vi "输入数据解析.vi"(0 "单个参数补充":dbl, 1 "从板号":dbl=1.0, 2 "主板二维码":string="BNET01", 3 "从板二维码":string="BNET01", 5 "主板引用":refnum<vi>, 7 "从板引用":refnum<vi>, 9 "主板选项":string="三级故障阀值", 11 "枚举":enum16{"主板", "从板"}(ring), 12 "快换":bool caption="快换写入") -> (4 "输出数组":dbl[][](array[numeric]), 6 "数组长度":dbl[](array[numeric]), 8 "循环次数":i32, 10 "命令":u32, 14 "名称":string[](array[string]), 15 "命令序号":u32[](array[numeric]))   [LabVIEW 2013] (continued)
                n2887 = Build Array(w7428, w7426) -> (w7429:i32[])
              }
            }
            n2888 = Insert Into Array(array=w7234, new element=w7235) -> (w7233:dbl[])  [unwired: 1 in]
          }
          n2889 = Build Array(w7230) -> (w7229:dbl[][])
          n2890 = Build Array("一级故障阀值") -> (w7220:string[])
        }
        frame "充电电流过高(2)" {
          n2891 = Unbundle By Name(w7455) -> ("一级故障 2"=w7456:refnum<vi>)
          n2892 = property class="Clust (严格)"(reference=w7456) -> ("Value"=w7454:T4)  [unwired: 1 in, 2 out]
          n2893 = for {
            N: 17 -> [_]
            tunnel: w7454 -> [w7466]
            shift-right: [w7463] -> w7460
            shift-left: dbl[] [] -> [w7464]
            i -> [w7467]
            n2894 = case shown="13" w7467 {
              tunnel: w7466 -> [w7468 w7479 w7490 w7500 w7510 w7520 w7532 w7544 w7556 w7568 w7580 w7592 w7606 w7627 w7639 w7648 w7657]
              tunnel: [w7469 w7480 w7491 w7501 w7511 w7522 w7534 w7546 w7558 w7570 w7582 w7593 w7615 w7630 w7638 w7647 w7659] -> w7465
              frame 0, Default {
                # "总电压过高"
                n2895 = disable-structure shown="启用" {
                  disable-tunnel: [w7475 w7478] -> w7471
                  disable-tunnel: [w7474 w7478] -> w7470
                  disable-tunnel: w7468 -> [w7473 _]
                  frame Disabled {
                    n2896 = Unbundle By Name(w7473) -> ("总电压过高"=w7472:dbl)
                    n2897 = call "输入分辨率计算-EV05.vi"("1字节?"=FALSE, "数值"=w7472, "分辨率"=0.1) -> ("低字节"=w7475:dbl, "高字节1"=w7474:dbl)  [unwired: 2 in, 5 out]
                  }
                  frame Enabled {
                    w7478 = 255 ("高字节1")
                  }
                }
                n2898 = Build Array(w7470, w7471) -> (w7469:i32[])
              }
              frame 1 {
                # "总电压过低"
                n2899 = disable-structure shown="启用" {
                  disable-tunnel: [w7486 w7489] -> w7482
                  disable-tunnel: [w7485 w7489] -> w7481
                  disable-tunnel: w7479 -> [w7484 _]
                  frame Disabled {
                    n2900 = Unbundle By Name(w7484) -> ("总电压过低"=w7483:dbl)
                    n2901 = call "输入分辨率计算-EV05.vi"("1字节?"=FALSE, "数值"=w7483, "分辨率"=0.1) -> ("低字节"=w7486:dbl, "高字节1"=w7485:dbl)  [unwired: 2 in, 5 out]
                  }
                  frame Enabled {
                    w7489 = 255 ("高字节1")
                  }
                }
                n2902 = Build Array(w7481, w7482) -> (w7480:i32[])
              }
              frame 2 {
                # "温度过高"
                n2903 = disable-structure shown="启用" {
                  disable-tunnel: [w7496 255 ("高字节1")] -> w7492
                  disable-tunnel: w7490 -> [w7494 _]
                  frame Disabled {
                    n2904 = Unbundle By Name(w7494) -> ("温度过高"=w7493:dbl)
                    n2905 = call "输入分辨率计算-EV05.vi"("1字节?"=TRUE, "数值"=w7493, "偏移量"=-40.0, "分辨率"=1.0) -> ("高字节1"=w7496:dbl)  [unwired: 1 in, 6 out]
                  }
                  frame Enabled {
                  }
                }
                n2906 = Build Array(w7492) -> (w7491:i32[])
              }
              frame 3 {
                # "温度过低"
                n2907 = disable-structure shown="启用" {
                  disable-tunnel: [w7506 255 ("高字节1")] -> w7502
                  disable-tunnel: w7500 -> [w7504 _]
                  frame Disabled {
                    n2908 = Unbundle By Name(w7504) -> ("温度过低"=w7503:dbl)
                    n2909 = call "输入分辨率计算-EV05.vi"("1字节?"=TRUE, "数值"=w7503, "偏移量"=-40.0, "分辨率"=1.0) -> ("高字节1"=w7506:dbl)  [unwired: 1 in, 6 out]
                  }
                  frame Enabled {
                  }
                }
                n2910 = Build Array(w7502) -> (w7501:i32[])
              }
              frame 4 {
                # "整组温度不均衡"
                n2911 = disable-structure shown="启用" {
                  disable-tunnel: [w7516 255 ("高字节1")] -> w7512
                  disable-tunnel: w7510 -> [w7514 _]
                  frame Disabled {
                    n2912 = Unbundle By Name(w7514) -> ("整组温度不均衡"=w7513:dbl)
                    n2913 = call "输入分辨率计算-EV05.vi"("1字节?"=TRUE, "数值"=w7513, "偏移量"=0.0, "分辨率"=1.0) -> ("高字节1"=w7516:dbl)  [unwired: 1 in, 6 out]
                  }
                  frame Enabled {
                  }
                }
                n2914 = Build Array(w7512) -> (w7511:i32[])
              }
              frame 5 {
                # "单组电压不均衡"
                n2915 = disable-structure shown="启用" {
                  disable-tunnel: [w7528 w7531] -> w7523
                  disable-tunnel: [w7526 w7531] -> w7521
                  disable-tunnel: w7520 -> [w7525 _]
                  frame Disabled {
                    n2916 = Unbundle By Name(w7525) -> ("单组电压不均衡"=w7524:dbl)
                    n2917 = call "输入分辨率计算-EV05.vi"("1字节?"=FALSE, "数值"=w7524, "偏移量"=0.0, "分辨率"=0.001) -> ("低字节"=w7526:dbl, "高字节1"=w7528:dbl)  [unwired: 1 in, 5 out]
                  }
                  frame Enabled {
                    w7531 = 255 ("高字节1")
                  }
                }
                n2918 = Build Array(w7523, w7521) -> (w7522:i32[])
              }
              frame 6 {
                # "整组电压不均衡"
                n2919 = disable-structure shown="启用" {
                  disable-tunnel: [w7540 w7543] -> w7535
                  disable-tunnel: [w7538 w7543] -> w7533
                  disable-tunnel: w7532 -> [w7537 _]
                  frame Disabled {
                    n2920 = Unbundle By Name(w7537) -> ("整组电压不均衡"=w7536:dbl)
                    n2921 = call "输入分辨率计算-EV05.vi"("1字节?"=FALSE, "数值"=w7536, "偏移量"=0.0, "分辨率"=0.001) -> ("低字节"=w7538:dbl, "高字节1"=w7540:dbl)  [unwired: 1 in, 5 out]
                  }
                  frame Enabled {
                    w7543 = 255 ("高字节1")
                  }
                }
                n2922 = Build Array(w7535, w7533) -> (w7534:i32[])
              }
              frame 7 {
                # "单体电压过高"
                n2923 = disable-structure shown="启用" {
                  disable-tunnel: [w7552 w7555] -> w7547
                  disable-tunnel: [w7550 w7555] -> w7545
                  disable-tunnel: w7544 -> [w7549 _]
                  frame Disabled {
                    n2924 = Unbundle By Name(w7549) -> ("单体电压过高"=w7548:dbl)
                    n2925 = call "输入分辨率计算-EV05.vi"("1字节?"=FALSE, "数值"=w7548, "偏移量"=0.0, "分辨率"=0.001) -> ("低字节"=w7550:dbl, "高字节1"=w7552:dbl)  [unwired: 1 in, 5 out]
                  }
                  frame Enabled {
                    w7555 = 255 ("高字节1")
                  }
                }
                n2926 = Build Array(w7547, w7545) -> (w7546:i32[])
              }
              frame 8 {
                # "单体电压过低"
                n2927 = disable-structure shown="启用" {
                  disable-tunnel: [w7564 w7567] -> w7559
                  disable-tunnel: [w7562 w7567] -> w7557
                  disable-tunnel: w7556 -> [w7561 _]
                  frame Disabled {
                    n2928 = Unbundle By Name(w7561) -> ("单体电压过低"=w7560:dbl)
                    n2929 = call "输入分辨率计算-EV05.vi"("1字节?"=FALSE, "数值"=w7560, "偏移量"=0.0, "分辨率"=0.001) -> ("低字节"=w7562:dbl, "高字节1"=w7564:dbl)  [unwired: 1 in, 5 out]
                  }
                  frame Enabled {
                    w7567 = 255 ("高字节1")
                  }
                }
                n2930 = Build Array(w7559, w7557) -> (w7558:i32[])
              }
              frame 9 {
                # "充电电流过高"
                n2931 = disable-structure shown="启用" {
                  disable-tunnel: [w7576 w7579] -> w7571
                  disable-tunnel: [w7574 w7579] -> w7569
                  disable-tunnel: w7568 -> [w7573 _]
                  frame Enabled {
                    n2932 = Unbundle By Name(w7573) -> ("充电电流过高"=w7572:dbl)
                    n2933 = call "输入分辨率计算-EV05.vi"("1字节?"=FALSE, "数值"=w7572, "偏移量"=0.0, "分辨率"=0.1) -> ("低字节"=w7574:dbl, "高字节1"=w7576:dbl)  [unwired: 1 in, 5 out]
                  }
                  frame Disabled {
                    w7579 = 255 ("高字节1")
                  }
                }
                n2934 = Build Array(w7571, w7569) -> (w7570:dbl[])
              }
              frame 10 {
                # "放电电流过高"
                n2935 = disable-structure shown="启用" {
                  disable-tunnel: [w7588 w7591] -> w7583
                  disable-tunnel: [w7586 w7591] -> w7581
                  disable-tunnel: w7580 -> [w7585 _]
                  frame Disabled {
                    n2936 = Unbundle By Name(w7585) -> ("放电电流过高"=w7584:dbl)
                    n2937 = call "输入分辨率计算-EV05.vi"("1字节?"=FALSE, "数值"=w7584, "偏移量"=-3000.0, "分辨率"=0.1) -> ("低字节"=w7586:dbl, "高字节1"=w7588:dbl)  [unwired: 1 in, 5 out]
                  }
                  frame Enabled {
                    w7591 = 255 ("高字节1")
                  }
                }
                n2938 = Build Array(w7583, w7581) -> (w7582:i32[])
              }
              frame 11 {
                # "单组温度不均衡"
                n2939 = disable-structure shown="启用" {
                  disable-tunnel: [w7598 255 ("高字节1")] -> w7594
                  disable-tunnel: w7592 -> [w7596 _]
                  frame Disabled {
                    n2940 = Unbundle By Name(w7596) -> ("单组温度不均衡"=w7595:dbl)
                    n2941 = call "输入分辨率计算-EV05.vi"("1字节?"=TRUE, "数值"=w7595, "偏移量"=0.0, "分辨率"=1.0) -> ("高字节1"=w7598:dbl)  [unwired: 1 in, 6 out]
                  }
                  frame Enabled {
                  }
                }
                n2942 = Build Array(w7594) -> (w7593:i32[])
              }
              frame 12 {
                # "SOC过高"
                n2943 = Unbundle By Name(w7606) -> ("SOC过高"=w7605:dbl)
                n2944 = call "输入分辨率计算-EV05.vi"("1字节?"=FALSE, "数值"=w7605, "偏移量"=0.0, "分辨率"=0.1) -> ("低字节"=w7607:dbl, "高字节1"=w7608:dbl)  [unwired: 1 in, 5 out]
                n2945 = call "二进制解析-8.6.vi"("索引"=4, "数值"=w7608) -> ("低位子数组"=w7611:i32[])  [unwired: 3 out]
                n2946 = call "二进制解析-8.6.vi"("索引"=4, "数值"=w7607) -> ("低位子数组"=w7603:i32[], "高位子数组"=w7610:i32[])  [unwired: 2 out]
                n2947 = Insert Into Array(array=w7611, new element=w7610) -> (w7609:i32[])  [unwired: 1 in]
                n2948 = call "数值二进制转十进制-8.6.vi"("子数组"=w7609) -> ("十进制数值"=w7604:i32)  [unwired: 4 out]
                n2949 = disable-structure shown="启用" {
                  disable-tunnel: w7604 -> [w7619 _]
                  disable-tunnel: [w7619 255 ("高字节1")] -> w7602
                  disable-tunnel: [w7618 i32[] [] ("低位子数组 27")] -> _
                  disable-tunnel: w7603 -> [w7618 _]
                  frame Disabled {
                  }
                  frame Enabled {
                  }
                }
                n2950 = Build Array(w7602, w7602) -> (w7615:i32[])
              }
              frame 13 {
                # "SOC过低"
                n2951 = Unbundle By Name(w7627) -> ("SOC过低"=w7626:dbl)
                n2952 = call "输入分辨率计算-EV05.vi"("1字节?"=FALSE, "数值"=w7626, "偏移量"=0.0, "分辨率"=0.1) -> ("低字节"=w7624:dbl, "高字节1"=w7625:dbl)  [unwired: 1 in, 5 out]
                n2953 = call "二进制解析-8.6.vi"("索引"=4, "数值"=w7625) -> ("低位子数组"=w7623:i32[])  [unwired: 3 out]
                n2954 = disable-structure shown="启用" {
                  disable-tunnel: w7624 -> [w7634 _]
                  disable-tunnel: [w7634 255 ("高字节1")] -> w7622
                  disable-tunnel: w7623 -> [w7633 _]
                  disable-tunnel: [w7633 i32[] [] ("低位子数组")] -> _
                  frame Disabled {
                    (unwired) i32[] [] ("低位子数组 4")
                  }
                  frame Enabled {
                  }
                }
                n2955 = Build Array(w7622, w7622) -> (w7630:i32[])
              }
              frame 14 {
                # "内阻过大"
                n2956 = disable-structure shown="启用" {
                  disable-tunnel: w7639 -> [w7644 _]
                  disable-tunnel: [w7640 255 ("高字节1")] -> w7637
                  frame Disabled {
                    n2957 = Unbundle By Name(w7644) -> ("内阻过大"=w7643:dbl)
                    n2958 = call "输入分辨率计算-EV05.vi"("1字节?"=TRUE, "数值"=w7643, "分辨率"=0.1) -> ("高字节1"=w7640:dbl)  [unwired: 2 in, 6 out]
                  }
                  frame Enabled {
                  }
                }
                n2959 = Build Array(w7637) -> (w7638:i32[])
              }
              frame 15 {
                # "极柱温度过高"
                n2960 = disable-structure shown="启用" {
                  disable-tunnel: w7648 -> [w7654 _]
                  disable-tunnel: [w7650 255 ("高字节1")] -> w7646
                  frame Disabled {
                    n2961 = Unbundle By Name(w7654) -> ("极柱温度过高"=w7653:dbl)
                    n2962 = call "输入分辨率计算-EV05.vi"("1字节?"=TRUE, "数值"=w7653, "偏移量"=-40.0, "分辨率"=1.0) -> ("高字节1"=w7650:dbl)  [unwired: 1 in, 6 out]
                  }
                  frame Enabled {
                  }
                }
                n2963 = Build Array(w7646) -> (w7647:i32[])
              }
              frame 16 {
                # "SOH过低"
                n2964 = disable-structure shown="启用" {
                  disable-tunnel: [w7671 w7679] -> w7658
                  disable-tunnel: w7657 -> [w7668 _]
                  disable-tunnel: [w7660 w7679] -> w7656
                  frame Disabled {
                    n2965 = Unbundle By Name(w7668) -> ("SOH过低"=w7667:dbl)
                    n2966 = call "输入分辨率计算-EV05.vi"("1字节?"=FALSE, "数值"=w7667, "偏移量"=0.0, "分辨率"=0.1) -> ("低字节"=w7669:dbl, "高字节1"=w7670:dbl)  [unwired: 1 in, 5 out]
                    n2967 = call "二进制解析-8.6.vi"("索引"=4, "数值"=w7670) -> ("低位子数组"=w7673:i32[])  [unwired: 3 out]
                    n2968 = call "二进制解析-8.6.vi"("索引"=4, "数值"=w7669) -> ("低位子数组"=w7662:i32[], "高位子数组"=w7672:i32[])  [unwired: 2 out]
                    n2969 = call "二进制解析-8.6.vi"("索引"=4, "数值"=0) -> ("低位子数组"=w7663:i32[])  [unwired: 3 out]
                    n2970 = Insert Into Array(array=w7673, new element=w7672) -> (w7666:i32[])  [unwired: 1 in]
                    n2971 = Insert Into Array(array=w7662, new element=w7663) -> (w7661:i32[])  [unwired: 1 in]
                    n2972 = call "数值二进制转十进制-8.6.vi"("子数组"=w7666) -> ("十进制数值"=w7671:i32)  [unwired: 4 out]
                    n2973 = call "数值二进制转十进制-8.6.vi"("子数组"=w7661) -> ("十进制数值"=w7660:i32)  [unwired: 4 out]
                  }
                  frame Enabled {
                    w7679 = 255 ("高字节1")
                  }
                }
                n2974 = Build Array(w7658, w7656) -> (w7659:i32[])
              }
            }
            n2975 = Insert Into Array(array=w7464, new element=w7465) -> (w7463:dbl[])  [unwired: 1 in]
          }
          n2976 = Build Array(w7460) -> (w7459:dbl[][])
          n2977 = Build Array("二级故障阀值") -> (w7450:string[])
        }
        frame "充电电流过高(3)" {
          n2978 = Unbundle By Name(w7685) -> ("一级故障 3"=w7686:refnum<vi>)
          n2979 = property class="Clust (严格)"(reference=w7686) -> ("Value"=w7684:T4)  [unwired: 1 in, 2 out]
          n2980 = for {
            N: 17 -> [_]
            tunnel: w7684 -> [w7696]
            shift-right: [w7693] -> w7690
            shift-left: dbl[] [] -> [w7694]
            i -> [w7697]
            n2981 = case shown="13" w7697 {
              tunnel: w7696 -> [w7698 w7709 w7720 w7730 w7740 w7750 w7762 w7774 w7786 w7798 w7810 w7822 w7836 w7857 w7869 w7878 w7887]
              tunnel: [w7699 w7710 w7721 w7731 w7741 w7752 w7764 w7776 w7788 w7800 w7812 w7823 w7845 w7860 w7868 w7877 w7889] -> w7695
              frame 0, Default {
                # "总电压过高"
                n2982 = disable-structure shown="启用" {
                  disable-tunnel: [w7705 w7708] -> w7701
                  disable-tunnel: [w7704 w7708] -> w7700
                  disable-tunnel: w7698 -> [w7703 _]
                  frame Disabled {
                    n2983 = Unbundle By Name(w7703) -> ("总电压过高"=w7702:dbl)
                    n2984 = call "输入分辨率计算-EV05.vi"("1字节?"=FALSE, "数值"=w7702, "分辨率"=0.1) -> ("低字节"=w7705:dbl, "高字节1"=w7704:dbl)  [unwired: 2 in, 5 out]
                  }
                  frame Enabled {
                    w7708 = 255 ("高字节1")
                  }
                }
                n2985 = Build Array(w7700, w7701) -> (w7699:i32[])
              }
              frame 1 {
                # "总电压过低"
                n2986 = disable-structure shown="启用" {
                  disable-tunnel: [w7716 w7719] -> w7712
                  disable-tunnel: [w7715 w7719] -> w7711
                  disable-tunnel: w7709 -> [w7714 _]
                  frame Disabled {
                    n2987 = Unbundle By Name(w7714) -> ("总电压过低"=w7713:dbl)
                    n2988 = call "输入分辨率计算-EV05.vi"("1字节?"=FALSE, "数值"=w7713, "分辨率"=0.1) -> ("低字节"=w7716:dbl, "高字节1"=w7715:dbl)  [unwired: 2 in, 5 out]
                  }
                  frame Enabled {
                    w7719 = 255 ("高字节1")
                  }
                }
                n2989 = Build Array(w7711, w7712) -> (w7710:i32[])
              }
              frame 2 {
                # "温度过高"
                n2990 = disable-structure shown="启用" {
                  disable-tunnel: [w7726 255 ("高字节1")] -> w7722
                  disable-tunnel: w7720 -> [w7724 _]
                  frame Disabled {
                    n2991 = Unbundle By Name(w7724) -> ("温度过高"=w7723:dbl)
                    n2992 = call "输入分辨率计算-EV05.vi"("1字节?"=TRUE, "数值"=w7723, "偏移量"=-40.0, "分辨率"=1.0) -> ("高字节1"=w7726:dbl)  [unwired: 1 in, 6 out]
                  }
                  frame Enabled {
                  }
                }
                n2993 = Build Array(w7722) -> (w7721:i32[])
              }
              frame 3 {
                # "温度过低"
                n2994 = disable-structure shown="启用" {
                  disable-tunnel: [w7736 255 ("高字节1")] -> w7732
                  disable-tunnel: w7730 -> [w7734 _]
                  frame Disabled {
                    n2995 = Unbundle By Name(w7734) -> ("温度过低"=w7733:dbl)
                    n2996 = call "输入分辨率计算-EV05.vi"("1字节?"=TRUE, "数值"=w7733, "偏移量"=-40.0, "分辨率"=1.0) -> ("高字节1"=w7736:dbl)  [unwired: 1 in, 6 out]
                  }
                  frame Enabled {
                  }
                }
                n2997 = Build Array(w7732) -> (w7731:i32[])
              }
              frame 4 {
                # "整组温度不均衡"
                n2998 = disable-structure shown="启用" {
                  disable-tunnel: [w7746 255 ("高字节1")] -> w7742
                  disable-tunnel: w7740 -> [w7744 _]
                  frame Disabled {
                    n2999 = Unbundle By Name(w7744) -> ("整组温度不均衡"=w7743:dbl)
                    n3000 = call "输入分辨率计算-EV05.vi"("1字节?"=TRUE, "数值"=w7743, "偏移量"=0.0, "分辨率"=1.0) -> ("高字节1"=w7746:dbl)  [unwired: 1 in, 6 out]
                  }
                  frame Enabled {
                  }
                }
                n3001 = Build Array(w7742) -> (w7741:i32[])
              }
              frame 5 {
                # "单组电压不均衡"
                n3002 = disable-structure shown="启用" {
                  disable-tunnel: [w7758 w7761] -> w7753
                  disable-tunnel: [w7756 w7761] -> w7751
                  disable-tunnel: w7750 -> [w7755 _]
                  frame Disabled {
                    n3003 = Unbundle By Name(w7755) -> ("单组电压不均衡"=w7754:dbl)
                    n3004 = call "输入分辨率计算-EV05.vi"("1字节?"=FALSE, "数值"=w7754, "偏移量"=0.0, "分辨率"=0.001) -> ("低字节"=w7756:dbl, "高字节1"=w7758:dbl)  [unwired: 1 in, 5 out]
                  }
                  frame Enabled {
                    w7761 = 255 ("高字节1")
                  }
                }
                n3005 = Build Array(w7753, w7751) -> (w7752:i32[])
              }
              frame 6 {
                # "整组电压不均衡"
                n3006 = disable-structure shown="启用" {
                  disable-tunnel: [w7770 w7773] -> w7765
                  disable-tunnel: [w7768 w7773] -> w7763
                  disable-tunnel: w7762 -> [w7767 _]
                  frame Disabled {
                    n3007 = Unbundle By Name(w7767) -> ("整组电压不均衡"=w7766:dbl)
                    n3008 = call "输入分辨率计算-EV05.vi"("1字节?"=FALSE, "数值"=w7766, "偏移量"=0.0, "分辨率"=0.001) -> ("低字节"=w7768:dbl, "高字节1"=w7770:dbl)  [unwired: 1 in, 5 out]
                  }
                  frame Enabled {
                    w7773 = 255 ("高字节1")
                  }
                }
                n3009 = Build Array(w7765, w7763) -> (w7764:i32[])
              }
              frame 7 {
                # "单体电压过高"
                n3010 = disable-structure shown="启用" {
                  disable-tunnel: [w7782 w7785] -> w7777
                  disable-tunnel: [w7780 w7785] -> w7775
                  disable-tunnel: w7774 -> [w7779 _]
                  frame Disabled {
                    n3011 = Unbundle By Name(w7779) -> ("单体电压过高"=w7778:dbl)
                    n3012 = call "输入分辨率计算-EV05.vi"("1字节?"=FALSE, "数值"=w7778, "偏移量"=0.0, "分辨率"=0.001) -> ("低字节"=w7780:dbl, "高字节1"=w7782:dbl)  [unwired: 1 in, 5 out]
                  }
                  frame Enabled {
                    w7785 = 255 ("高字节1")
                  }
                }
                n3013 = Build Array(w7777, w7775) -> (w7776:i32[])
              }
              frame 8 {
                # "单体电压过低"
                n3014 = disable-structure shown="启用" {
                  disable-tunnel: [w7794 w7797] -> w7789
                  disable-tunnel: [w7792 w7797] -> w7787
                  disable-tunnel: w7786 -> [w7791 _]
                  frame Disabled {
                    n3015 = Unbundle By Name(w7791) -> ("单体电压过低"=w7790:dbl)
                    n3016 = call "输入分辨率计算-EV05.vi"("1字节?"=FALSE, "数值"=w7790, "偏移量"=0.0, "分辨率"=0.001) -> ("低字节"=w7792:dbl, "高字节1"=w7794:dbl)  [unwired: 1 in, 5 out]
                  }
                  frame Enabled {
                    w7797 = 255 ("高字节1")
                  }
                }
                n3017 = Build Array(w7789, w7787) -> (w7788:i32[])
              }
              frame 9 {
                # "充电电流过高"
                n3018 = disable-structure shown="启用" {
                  disable-tunnel: [w7806 w7809] -> w7801
                  disable-tunnel: [w7804 w7809] -> w7799
                  disable-tunnel: w7798 -> [w7803 _]
                  frame Enabled {
                    n3019 = Unbundle By Name(w7803) -> ("充电电流过高"=w7802:dbl)
                    n3020 = call "输入分辨率计算-EV05.vi"("1字节?"=FALSE, "数值"=w7802, "偏移量"=0.0, "分辨率"=0.1) -> ("低字节"=w7804:dbl, "高字节1"=w7806:dbl)  [unwired: 1 in, 5 out]
                  }
                  frame Disabled {
                    w7809 = 255 ("高字节1")
                  }
                }
                n3021 = Build Array(w7801, w7799) -> (w7800:dbl[])
              }
              frame 10 {
                # "放电电流过高"
                n3022 = disable-structure shown="启用" {
                  disable-tunnel: [w7818 w7821] -> w7813
                  disable-tunnel: [w7816 w7821] -> w7811
                  disable-tunnel: w7810 -> [w7815 _]
                  frame Disabled {
                    n3023 = Unbundle By Name(w7815) -> ("放电电流过高"=w7814:dbl)
                    n3024 = call "输入分辨率计算-EV05.vi"("1字节?"=FALSE, "数值"=w7814, "偏移量"=-3000.0, "分辨率"=0.1) -> ("低字节"=w7816:dbl, "高字节1"=w7818:dbl)  [unwired: 1 in, 5 out]
                  }
                  frame Enabled {
                    w7821 = 255 ("高字节1")
                  }
                }
                n3025 = Build Array(w7813, w7811) -> (w7812:i32[])
              }
              frame 11 {
                # "单组温度不均衡"
                n3026 = disable-structure shown="启用" {
                  disable-tunnel: [w7828 255 ("高字节1")] -> w7824
                  disable-tunnel: w7822 -> [w7826 _]
                  frame Disabled {
                    n3027 = Unbundle By Name(w7826) -> ("单组温度不均衡"=w7825:dbl)
                    n3028 = call "输入分辨率计算-EV05.vi"("1字节?"=TRUE, "数值"=w7825, "偏移量"=0.0, "分辨率"=1.0) -> ("高字节1"=w7828:dbl)  [unwired: 1 in, 6 out]
                  }
                  frame Enabled {
                  }
                }
                n3029 = Build Array(w7824) -> (w7823:i32[])
              }
              frame 12 {
                # "SOC过高"
                n3030 = Unbundle By Name(w7836) -> ("SOC过高"=w7835:dbl)
                n3031 = call "输入分辨率计算-EV05.vi"("1字节?"=FALSE, "数值"=w7835, "偏移量"=0.0, "分辨率"=0.1) -> ("低字节"=w7837:dbl, "高字节1"=w7838:dbl)  [unwired: 1 in, 5 out]
                n3032 = call "二进制解析-8.6.vi"("索引"=4, "数值"=w7838) -> ("低位子数组"=w7841:i32[])  [unwired: 3 out]
                n3033 = call "二进制解析-8.6.vi"("索引"=4, "数值"=w7837) -> ("低位子数组"=w7833:i32[], "高位子数组"=w7840:i32[])  [unwired: 2 out]
                n3034 = Insert Into Array(array=w7841, new element=w7840) -> (w7839:i32[])  [unwired: 1 in]
                n3035 = call "数值二进制转十进制-8.6.vi"("子数组"=w7839) -> ("十进制数值"=w7834:i32)  [unwired: 4 out]
                n3036 = disable-structure shown="启用" {
                  disable-tunnel: w7834 -> [w7849 _]
                  disable-tunnel: [w7849 255 ("高字节1")] -> w7832
                  disable-tunnel: [w7848 i32[] [] ("低位子数组 27")] -> _
                  disable-tunnel: w7833 -> [w7848 _]
                  frame Disabled {
                  }
                  frame Enabled {
                  }
                }
                n3037 = Build Array(w7832, w7832) -> (w7845:i32[])
              }
              frame 13 {
                # "SOC过低"
                n3038 = Unbundle By Name(w7857) -> ("SOC过低"=w7856:dbl)
                n3039 = call "输入分辨率计算-EV05.vi"("1字节?"=FALSE, "数值"=w7856, "偏移量"=0.0, "分辨率"=0.1) -> ("低字节"=w7854:dbl, "高字节1"=w7855:dbl)  [unwired: 1 in, 5 out]
                n3040 = call "二进制解析-8.6.vi"("索引"=4, "数值"=w7855) -> ("低位子数组"=w7853:i32[])  [unwired: 3 out]
                n3041 = disable-structure shown="启用" {
                  disable-tunnel: w7854 -> [w7864 _]
                  disable-tunnel: [w7864 255 ("高字节1")] -> w7852
                  disable-tunnel: w7853 -> [w7863 _]
                  disable-tunnel: [w7863 i32[] [] ("低位子数组")] -> _
                  frame Disabled {
                    (unwired) i32[] [] ("低位子数组 4")
                  }
                  frame Enabled {
                  }
                }
                n3042 = Build Array(w7852, w7852) -> (w7860:i32[])
              }
              frame 14 {
                # "内阻过大"
                n3043 = disable-structure shown="启用" {
                  disable-tunnel: w7869 -> [w7874 _]
                  disable-tunnel: [w7870 255 ("高字节1")] -> w7867
                  frame Disabled {
                    n3044 = Unbundle By Name(w7874) -> ("内阻过大"=w7873:dbl)
                    n3045 = call "输入分辨率计算-EV05.vi"("1字节?"=TRUE, "数值"=w7873, "分辨率"=0.1) -> ("高字节1"=w7870:dbl)  [unwired: 2 in, 6 out]
                  }
                  frame Enabled {
                  }
                }
                n3046 = Build Array(w7867) -> (w7868:i32[])
              }
              frame 15 {
                # "极柱温度过高"
                n3047 = disable-structure shown="启用" {
                  disable-tunnel: w7878 -> [w7884 _]
                  disable-tunnel: [w7880 255 ("高字节1")] -> w7876
                  frame Disabled {
                    n3048 = Unbundle By Name(w7884) -> ("极柱温度过高"=w7883:dbl)
                    n3049 = call "输入分辨率计算-EV05.vi"("1字节?"=TRUE, "数值"=w7883, "偏移量"=-40.0, "分辨率"=1.0) -> ("高字节1"=w7880:dbl)  [unwired: 1 in, 6 out]
                  }
                  frame Enabled {
                  }
                }
                n3050 = Build Array(w7876) -> (w7877:i32[])
              }
              frame 16 {
                # "SOH过低"
                n3051 = disable-structure shown="启用" {
                  disable-tunnel: [w7901 w7909] -> w7888
                  disable-tunnel: w7887 -> [w7898 _]
                  disable-tunnel: [w7890 w7909] -> w7886
                  frame Disabled {
                    n3052 = Unbundle By Name(w7898) -> ("SOH过低"=w7897:dbl)
                    n3053 = call "输入分辨率计算-EV05.vi"("1字节?"=FALSE, "数值"=w7897, "偏移量"=0.0, "分辨率"=0.1) -> ("低字节"=w7899:dbl, "高字节1"=w7900:dbl)  [unwired: 1 in, 5 out]
                    n3054 = call "二进制解析-8.6.vi"("索引"=4, "数值"=w7900) -> ("低位子数组"=w7903:i32[])  [unwired: 3 out]
                    n3055 = call "二进制解析-8.6.vi"("索引"=4, "数值"=w7899) -> ("低位子数组"=w7892:i32[], "高位子数组"=w7902:i32[])  [unwired: 2 out]
                    n3056 = call "二进制解析-8.6.vi"("索引"=4, "数值"=0) -> ("低位子数组"=w7893:i32[])  [unwired: 3 out]
                    n3057 = Insert Into Array(array=w7903, new element=w7902) -> (w7896:i32[])  [unwired: 1 in]
                    n3058 = Insert Into Array(array=w7892, new element=w7893) -> (w7891:i32[])  [unwired: 1 in]
                    n3059 = call "数值二进制转十进制-8.6.vi"("子数组"=w7896) -> ("十进制数值"=w7901:i32)  [unwired: 4 out]
                    n3060 = call "数值二进制转十进制-8.6.vi"("子数组"=w7891) -> ("十进制数值"=w7890:i32)  [unwired: 4 out]
                  }
                  frame Enabled {
                    w7909 = 255 ("高字节1")
                  }
                }
                n3061 = Build Array(w7888, w7886) -> (w7889:i32[])
              }
            }
            n3062 = Insert Into Array(array=w7694, new element=w7695) -> (w7693:dbl[])  [unwired: 1 in]
          }
          n3063 = Build Array(w7690) -> (w7689:dbl[][])
          n3064 = Build Array("三级故障阀值") -> (w7680:string[])
        }
        frame "放电电流过高" {
          n3065 = Unbundle By Name(w7915) -> ("一级故障"=w7916:refnum<vi>)
          n3066 = property class="Clust (严格)"(reference=w7916) -> ("Value"=w7914:T4)  [unwired: 1 in, 2 out]
          n3067 = for {
            N: 17 -> [_]
            tunnel: w7914 -> [w7926]
            shift-right: [w7923] -> w7920
            shift-left: dbl[] [] -> [w7924]
            i -> [w7927]
            n3068 = case shown="14" w7927 {
              tunnel: w7926 -> [w7928 w7939 w7950 w7960 w7970 w7980 w7992 w8004 w8016 w8028 w8040 w8052 w8066 w8087 w8099 w8108 w8117]
              tunnel: [w7929 w7940 w7951 w7961 w7971 w7982 w7994 w8006 w8018 w8030 w8042 w8053 w8075 w8090 w8098 w8107 w8119] -> w7925
              frame 0, Default {
                # "总电压过高"
                n3069 = disable-structure shown="启用" {
                  disable-tunnel: [w7935 w7938] -> w7931
                  disable-tunnel: [w7934 w7938] -> w7930
                  disable-tunnel: w7928 -> [w7933 _]
                  frame Disabled {
                    n3070 = Unbundle By Name(w7933) -> ("总电压过高"=w7932:dbl)
                    n3071 = call "输入分辨率计算-EV05.vi"("1字节?"=FALSE, "数值"=w7932, "分辨率"=0.1) -> ("低字节"=w7935:dbl, "高字节1"=w7934:dbl)  [unwired: 2 in, 5 out]
                  }
                  frame Enabled {
                    w7938 = 255 ("高字节1")
                  }
                }
                n3072 = Build Array(w7930, w7931) -> (w7929:i32[])
              }
              frame 1 {
                # "总电压过低"
                n3073 = disable-structure shown="启用" {
                  disable-tunnel: [w7946 w7949] -> w7942
                  disable-tunnel: [w7945 w7949] -> w7941
                  disable-tunnel: w7939 -> [w7944 _]
                  frame Disabled {
                    n3074 = Unbundle By Name(w7944) -> ("总电压过低"=w7943:dbl)
                    n3075 = call "输入分辨率计算-EV05.vi"("1字节?"=FALSE, "数值"=w7943, "分辨率"=0.1) -> ("低字节"=w7946:dbl, "高字节1"=w7945:dbl)  [unwired: 2 in, 5 out]
                  }
                  frame Enabled {
                    w7949 = 255 ("高字节1")
                  }
                }
                n3076 = Build Array(w7941, w7942) -> (w7940:i32[])
              }
              frame 2 {
                # "温度过高"
                n3077 = disable-structure shown="启用" {
                  disable-tunnel: [w7956 255 ("高字节1")] -> w7952
                  disable-tunnel: w7950 -> [w7954 _]
                  frame Disabled {
                    n3078 = Unbundle By Name(w7954) -> ("温度过高"=w7953:dbl)
                    n3079 = call "输入分辨率计算-EV05.vi"("1字节?"=TRUE, "数值"=w7953, "偏移量"=-40.0, "分辨率"=1.0) -> ("高字节1"=w7956:dbl)  [unwired: 1 in, 6 out]
                  }
                  frame Enabled {
                  }
                }
                n3080 = Build Array(w7952) -> (w7951:i32[])
              }
              frame 3 {
                # "温度过低"
                n3081 = disable-structure shown="启用" {
                  disable-tunnel: [w7966 255 ("高字节1")] -> w7962
                  disable-tunnel: w7960 -> [w7964 _]
                  frame Disabled {
                    n3082 = Unbundle By Name(w7964) -> ("温度过低"=w7963:dbl)
                    n3083 = call "输入分辨率计算-EV05.vi"("1字节?"=TRUE, "数值"=w7963, "偏移量"=-40.0, "分辨率"=1.0) -> ("高字节1"=w7966:dbl)  [unwired: 1 in, 6 out]
                  }
                  frame Enabled {
                  }
                }
                n3084 = Build Array(w7962) -> (w7961:i32[])
              }
              frame 4 {
                # "整组温度不均衡"
                n3085 = disable-structure shown="启用" {
                  disable-tunnel: [w7976 255 ("高字节1")] -> w7972
                  disable-tunnel: w7970 -> [w7974 _]
                  frame Disabled {
                    n3086 = Unbundle By Name(w7974) -> ("整组温度不均衡"=w7973:dbl)
                    n3087 = call "输入分辨率计算-EV05.vi"("1字节?"=TRUE, "数值"=w7973, "偏移量"=0.0, "分辨率"=1.0) -> ("高字节1"=w7976:dbl)  [unwired: 1 in, 6 out]
                  }
                  frame Enabled {
                  }
                }
                n3088 = Build Array(w7972) -> (w7971:i32[])
              }
              frame 5 {
                # "单组电压不均衡"
                n3089 = disable-structure shown="启用" {
                  disable-tunnel: [w7988 w7991] -> w7983
                  disable-tunnel: [w7986 w7991] -> w7981
                  disable-tunnel: w7980 -> [w7985 _]
                  frame Disabled {
                    n3090 = Unbundle By Name(w7985) -> ("单组电压不均衡"=w7984:dbl)
                    n3091 = call "输入分辨率计算-EV05.vi"("1字节?"=FALSE, "数值"=w7984, "偏移量"=0.0, "分辨率"=0.001) -> ("低字节"=w7986:dbl, "高字节1"=w7988:dbl)  [unwired: 1 in, 5 out]
                  }
                  frame Enabled {
                    w7991 = 255 ("高字节1")
                  }
                }
                n3092 = Build Array(w7983, w7981) -> (w7982:i32[])
              }
              frame 6 {
                # "整组电压不均衡"
                n3093 = disable-structure shown="启用" {
                  disable-tunnel: [w8000 w8003] -> w7995
                  disable-tunnel: [w7998 w8003] -> w7993
                  disable-tunnel: w7992 -> [w7997 _]
                  frame Disabled {
                    n3094 = Unbundle By Name(w7997) -> ("整组电压不均衡"=w7996:dbl)
                    n3095 = call "输入分辨率计算-EV05.vi"("1字节?"=FALSE, "数值"=w7996, "偏移量"=0.0, "分辨率"=0.001) -> ("低字节"=w7998:dbl, "高字节1"=w8000:dbl)  [unwired: 1 in, 5 out]
                  }
                  frame Enabled {
                    w8003 = 255 ("高字节1")
                  }
                }
                n3096 = Build Array(w7995, w7993) -> (w7994:i32[])
              }
              frame 7 {
                # "单体电压过高"
                n3097 = disable-structure shown="启用" {
                  disable-tunnel: [w8012 w8015] -> w8007
                  disable-tunnel: [w8010 w8015] -> w8005
                  disable-tunnel: w8004 -> [w8009 _]
                  frame Disabled {
                    n3098 = Unbundle By Name(w8009) -> ("单体电压过高"=w8008:dbl)
                    n3099 = call "输入分辨率计算-EV05.vi"("1字节?"=FALSE, "数值"=w8008, "偏移量"=0.0, "分辨率"=0.001) -> ("低字节"=w8010:dbl, "高字节1"=w8012:dbl)  [unwired: 1 in, 5 out]
                  }
                  frame Enabled {
                    w8015 = 255 ("高字节1")
                  }
                }
                n3100 = Build Array(w8007, w8005) -> (w8006:i32[])
              }
              frame 8 {
                # "单体电压过低"
                n3101 = disable-structure shown="启用" {
                  disable-tunnel: [w8024 w8027] -> w8019
                  disable-tunnel: [w8022 w8027] -> w8017
                  disable-tunnel: w8016 -> [w8021 _]
                  frame Disabled {
                    n3102 = Unbundle By Name(w8021) -> ("单体电压过低"=w8020:dbl)
                    n3103 = call "输入分辨率计算-EV05.vi"("1字节?"=FALSE, "数值"=w8020, "偏移量"=0.0, "分辨率"=0.001) -> ("低字节"=w8022:dbl, "高字节1"=w8024:dbl)  [unwired: 1 in, 5 out]
                  }
                  frame Enabled {
                    w8027 = 255 ("高字节1")
                  }
                }
                n3104 = Build Array(w8019, w8017) -> (w8018:i32[])
              }
              frame 9 {
                # "充电电流过高"
                n3105 = disable-structure shown="启用" {
                  disable-tunnel: [w8036 w8039] -> w8031
                  disable-tunnel: [w8034 w8039] -> w8029
                  disable-tunnel: w8028 -> [w8033 _]
                  frame Disabled {
                    n3106 = Unbundle By Name(w8033) -> ("充电电流过高"=w8032:dbl)
                    n3107 = call "输入分辨率计算-EV05.vi"("1字节?"=FALSE, "数值"=w8032, "偏移量"=-3000.0, "分辨率"=0.1) -> ("低字节"=w8034:dbl, "高字节1"=w8036:dbl)  [unwired: 1 in, 5 out]
                  }
                  frame Enabled {
                    w8039 = 255 ("高字节1")
                  }
                }
                n3108 = Build Array(w8031, w8029) -> (w8030:i32[])
              }
              frame 10 {
                # "放电电流过高"
                n3109 = disable-structure shown="启用" {
                  disable-tunnel: [w8048 w8051] -> w8043
                  disable-tunnel: [w8046 w8051] -> w8041
                  disable-tunnel: w8040 -> [w8045 _]
                  frame Enabled {
                    n3110 = Unbundle By Name(w8045) -> ("放电电流过高"=w8044:dbl)
                    n3111 = call "输入分辨率计算-EV05.vi"("1字节?"=FALSE, "数值"=w8044, "偏移量"=0.0, "分辨率"=0.1) -> ("低字节"=w8046:dbl, "高字节1"=w8048:dbl)  [unwired: 1 in, 5 out]
                  }
                  frame Disabled {
                    w8051 = 255 ("高字节1")
                  }
                }
                n3112 = Build Array(w8043, w8041) -> (w8042:dbl[])
              }
              frame 11 {
                # "单组温度不均衡"
                n3113 = disable-structure shown="启用" {
                  disable-tunnel: [w8058 255 ("高字节1")] -> w8054
                  disable-tunnel: w8052 -> [w8056 _]
                  frame Disabled {
                    n3114 = Unbundle By Name(w8056) -> ("单组温度不均衡"=w8055:dbl)
                    n3115 = call "输入分辨率计算-EV05.vi"("1字节?"=TRUE, "数值"=w8055, "偏移量"=0.0, "分辨率"=1.0) -> ("高字节1"=w8058:dbl)  [unwired: 1 in, 6 out]
                  }
                  frame Enabled {
                  }
                }
                n3116 = Build Array(w8054) -> (w8053:i32[])
              }
              frame 12 {
                # "SOC过高"
                n3117 = Unbundle By Name(w8066) -> ("SOC过高"=w8065:dbl)
                n3118 = call "输入分辨率计算-EV05.vi"("1字节?"=FALSE, "数值"=w8065, "偏移量"=0.0, "分辨率"=0.1) -> ("低字节"=w8067:dbl, "高字节1"=w8068:dbl)  [unwired: 1 in, 5 out]
                n3119 = call "二进制解析-8.6.vi"("索引"=4, "数值"=w8068) -> ("低位子数组"=w8071:i32[])  [unwired: 3 out]
                n3120 = call "二进制解析-8.6.vi"("索引"=4, "数值"=w8067) -> ("低位子数组"=w8063:i32[], "高位子数组"=w8070:i32[])  [unwired: 2 out]
                n3121 = Insert Into Array(array=w8071, new element=w8070) -> (w8069:i32[])  [unwired: 1 in]
                n3122 = call "数值二进制转十进制-8.6.vi"("子数组"=w8069) -> ("十进制数值"=w8064:i32)  [unwired: 4 out]
                n3123 = disable-structure shown="启用" {
                  disable-tunnel: w8064 -> [w8079 _]
                  disable-tunnel: [w8079 255 ("高字节1")] -> w8062
                  disable-tunnel: [w8078 i32[] [] ("低位子数组 28")] -> _
                  disable-tunnel: w8063 -> [w8078 _]
                  frame Disabled {
                  }
                  frame Enabled {
                  }
                }
                n3124 = Build Array(w8062, w8062) -> (w8075:i32[])
              }
              frame 13 {
                # "SOC过低"
                n3125 = Unbundle By Name(w8087) -> ("SOC过低"=w8086:dbl)
                n3126 = call "输入分辨率计算-EV05.vi"("1字节?"=FALSE, "数值"=w8086, "偏移量"=0.0, "分辨率"=0.1) -> ("低字节"=w8084:dbl, "高字节1"=w8085:dbl)  [unwired: 1 in, 5 out]
                n3127 = call "二进制解析-8.6.vi"("索引"=4, "数值"=w8085) -> ("低位子数组"=w8083:i32[])  [unwired: 3 out]
                n3128 = disable-structure shown="启用" {
                  disable-tunnel: w8084 -> [w8094 _]
                  disable-tunnel: [w8094 255 ("高字节1")] -> w8082
                  disable-tunnel: w8083 -> [w8093 _]
                  disable-tunnel: [w8093 i32[] [] ("低位子数组")] -> _
                  frame Disabled {
                    (unwired) i32[] [] ("低位子数组 4")
                  }
                  frame Enabled {
                  }
                }
                n3129 = Build Array(w8082, w8082) -> (w8090:i32[])
              }
              frame 14 {
                # "内阻过大"
                n3130 = disable-structure shown="启用" {
                  disable-tunnel: w8099 -> [w8104 _]
                  disable-tunnel: [w8100 255 ("高字节1")] -> w8097
                  frame Disabled {
                    n3131 = Unbundle By Name(w8104) -> ("内阻过大"=w8103:dbl)
                    n3132 = call "输入分辨率计算-EV05.vi"("1字节?"=TRUE, "数值"=w8103, "分辨率"=0.1) -> ("高字节1"=w8100:dbl)  [unwired: 2 in, 6 out]
                  }
                  frame Enabled {
                  }
                }
                n3133 = Build Array(w8097) -> (w8098:i32[])
              }
              frame 15 {
                # "极柱温度过高"
                n3134 = disable-structure shown="启用" {
                  disable-tunnel: w8108 -> [w8114 _]
                  disable-tunnel: [w8110 255 ("高字节1")] -> w8106
                  frame Disabled {
                    n3135 = Unbundle By Name(w8114) -> ("极柱温度过高"=w8113:dbl)
                    n3136 = call "输入分辨率计算-EV05.vi"("1字节?"=TRUE, "数值"=w8113, "偏移量"=-40.0, "分辨率"=1.0) -> ("高字节1"=w8110:dbl)  [unwired: 1 in, 6 out]
                  }
                  frame Enabled {
                  }
                }
                n3137 = Build Array(w8106) -> (w8107:i32[])
              }
              frame 16 {
                # "SOH过低"
                n3138 = disable-structure shown="启用" {
                  disable-tunnel: [w8131 w8139] -> w8118
                  disable-tunnel: w8117 -> [w8128 _]
                  disable-tunnel: [w8120 w8139] -> w8116
                  frame Disabled {
                    n3139 = Unbundle By Name(w8128) -> ("SOH过低"=w8127:dbl)
                    n3140 = call "输入分辨率计算-EV05.vi"("1字节?"=FALSE, "数值"=w8127, "偏移量"=0.0, "分辨率"=0.1) -> ("低字节"=w8129:dbl, "高字节1"=w8130:dbl)  [unwired: 1 in, 5 out]
                    n3141 = call "二进制解析-8.6.vi"("索引"=4, "数值"=w8130) -> ("低位子数组"=w8133:i32[])  [unwired: 3 out]
                    n3142 = call "二进制解析-8.6.vi"("索引"=4, "数值"=w8129) -> ("低位子数组"=w8122:i32[], "高位子数组"=w8132:i32[])  [unwired: 2 out]
                    n3143 = call "二进制解析-8.6.vi"("索引"=4, "数值"=0) -> ("低位子数组"=w8123:i32[])  [unwired: 3 out]
                    n3144 = Insert Into Array(array=w8133, new element=w8132) -> (w8126:i32[])  [unwired: 1 in]
                    n3145 = Insert Into Array(array=w8122, new element=w8123) -> (w8121:i32[])  [unwired: 1 in]
                    n3146 = call "数值二进制转十进制-8.6.vi"("子数组"=w8126) -> ("十进制数值"=w8131:i32)  [unwired: 4 out]
                    n3147 = call "数值二进制转十进制-8.6.vi"("子数组"=w8121) -> ("十进制数值"=w8120:i32)  [unwired: 4 out]
                  }
                  frame Enabled {
                    w8139 = 255 ("高字节1")
                  }
                }
                n3148 = Build Array(w8118, w8116) -> (w8119:i32[])
              }
            }
            n3149 = Insert Into Array(array=w7924, new element=w7925) -> (w7923:dbl[])  [unwired: 1 in]
          }
          n3150 = Build Array(w7920) -> (w7919:dbl[][])
          n3151 = Build Array("一级故障阀值") -> (w7910:string[])
        }
        frame "放电电流过高(2)" {
          n3152 = Unbundle By Name(w8145) -> ("一级故障 2"=w8146:refnum<vi>)
          n3153 = property class="Clust (严格)"(reference=w8146) -> ("Value"=w8144:T4)  [unwired: 1 in, 2 out]
          n3154 = for {
            N: 17 -> [_]
            tunnel: w8144 -> [w8156]
            shift-right: [w8153] -> w8150
            shift-left: dbl[] [] -> [w8154]
            i -> [w8157]
            n3155 = case shown="12" w8157 {
              tunnel: w8156 -> [w8158 w8169 w8180 w8190 w8200 w8210 w8222 w8234 w8246 w8258 w8270 w8282 w8296 w8317 w8329 w8338 w8347]
              tunnel: [w8159 w8170 w8181 w8191 w8201 w8212 w8224 w8236 w8248 w8260 w8272 w8283 w8305 w8320 w8328 w8337 w8349] -> w8155
              frame 0, Default {
                # "总电压过高"
                n3156 = disable-structure shown="启用" {
                  disable-tunnel: [w8165 w8168] -> w8161
                  disable-tunnel: [w8164 w8168] -> w8160
                  disable-tunnel: w8158 -> [w8163 _]
                  frame Disabled {
                    n3157 = Unbundle By Name(w8163) -> ("总电压过高"=w8162:dbl)
                    n3158 = call "输入分辨率计算-EV05.vi"("1字节?"=FALSE, "数值"=w8162, "分辨率"=0.1) -> ("低字节"=w8165:dbl, "高字节1"=w8164:dbl)  [unwired: 2 in, 5 out]
                  }
                  frame Enabled {
                    w8168 = 255 ("高字节1")
                  }
                }
                n3159 = Build Array(w8160, w8161) -> (w8159:i32[])
              }
              frame 1 {
                # "总电压过低"
                n3160 = disable-structure shown="启用" {
                  disable-tunnel: [w8176 w8179] -> w8172
                  disable-tunnel: [w8175 w8179] -> w8171
                  disable-tunnel: w8169 -> [w8174 _]
                  frame Disabled {
                    n3161 = Unbundle By Name(w8174) -> ("总电压过低"=w8173:dbl)
                    n3162 = call "输入分辨率计算-EV05.vi"("1字节?"=FALSE, "数值"=w8173, "分辨率"=0.1) -> ("低字节"=w8176:dbl, "高字节1"=w8175:dbl)  [unwired: 2 in, 5 out]
                  }
                  frame Enabled {
                    w8179 = 255 ("高字节1")
                  }
                }
                n3163 = Build Array(w8171, w8172) -> (w8170:i32[])
              }
              frame 2 {
                # "温度过高"
                n3164 = disable-structure shown="启用" {
                  disable-tunnel: [w8186 255 ("高字节1")] -> w8182
                  disable-tunnel: w8180 -> [w8184 _]
                  frame Disabled {
                    n3165 = Unbundle By Name(w8184) -> ("温度过高"=w8183:dbl)
                    n3166 = call "输入分辨率计算-EV05.vi"("1字节?"=TRUE, "数值"=w8183, "偏移量"=-40.0, "分辨率"=1.0) -> ("高字节1"=w8186:dbl)  [unwired: 1 in, 6 out]
                  }
                  frame Enabled {
                  }
                }
                n3167 = Build Array(w8182) -> (w8181:i32[])
              }
              frame 3 {
                # "温度过低"
                n3168 = disable-structure shown="启用" {
                  disable-tunnel: [w8196 255 ("高字节1")] -> w8192
                  disable-tunnel: w8190 -> [w8194 _]
                  frame Disabled {
                    n3169 = Unbundle By Name(w8194) -> ("温度过低"=w8193:dbl)
                    n3170 = call "输入分辨率计算-EV05.vi"("1字节?"=TRUE, "数值"=w8193, "偏移量"=-40.0, "分辨率"=1.0) -> ("高字节1"=w8196:dbl)  [unwired: 1 in, 6 out]
                  }
                  frame Enabled {
                  }
                }
                n3171 = Build Array(w8192) -> (w8191:i32[])
              }
              frame 4 {
                # "整组温度不均衡"
                n3172 = disable-structure shown="启用" {
                  disable-tunnel: [w8206 255 ("高字节1")] -> w8202
                  disable-tunnel: w8200 -> [w8204 _]
                  frame Disabled {
                    n3173 = Unbundle By Name(w8204) -> ("整组温度不均衡"=w8203:dbl)
                    n3174 = call "输入分辨率计算-EV05.vi"("1字节?"=TRUE, "数值"=w8203, "偏移量"=0.0, "分辨率"=1.0) -> ("高字节1"=w8206:dbl)  [unwired: 1 in, 6 out]
                  }
                  frame Enabled {
                  }
                }
                n3175 = Build Array(w8202) -> (w8201:i32[])
              }
              frame 5 {
                # "单组电压不均衡"
                n3176 = disable-structure shown="启用" {
                  disable-tunnel: [w8218 w8221] -> w8213
                  disable-tunnel: [w8216 w8221] -> w8211
                  disable-tunnel: w8210 -> [w8215 _]
                  frame Disabled {
                    n3177 = Unbundle By Name(w8215) -> ("单组电压不均衡"=w8214:dbl)
                    n3178 = call "输入分辨率计算-EV05.vi"("1字节?"=FALSE, "数值"=w8214, "偏移量"=0.0, "分辨率"=0.001) -> ("低字节"=w8216:dbl, "高字节1"=w8218:dbl)  [unwired: 1 in, 5 out]
                  }
                  frame Enabled {
                    w8221 = 255 ("高字节1")
                  }
                }
                n3179 = Build Array(w8213, w8211) -> (w8212:i32[])
              }
              frame 6 {
                # "整组电压不均衡"
                n3180 = disable-structure shown="启用" {
                  disable-tunnel: [w8230 w8233] -> w8225
                  disable-tunnel: [w8228 w8233] -> w8223
                  disable-tunnel: w8222 -> [w8227 _]
                  frame Disabled {
                    n3181 = Unbundle By Name(w8227) -> ("整组电压不均衡"=w8226:dbl)
                    n3182 = call "输入分辨率计算-EV05.vi"("1字节?"=FALSE, "数值"=w8226, "偏移量"=0.0, "分辨率"=0.001) -> ("低字节"=w8228:dbl, "高字节1"=w8230:dbl)  [unwired: 1 in, 5 out]
                  }
                  frame Enabled {
                    w8233 = 255 ("高字节1")
                  }
                }
                n3183 = Build Array(w8225, w8223) -> (w8224:i32[])
              }
              frame 7 {
                # "单体电压过高"
                n3184 = disable-structure shown="启用" {
                  disable-tunnel: [w8242 w8245] -> w8237
                  disable-tunnel: [w8240 w8245] -> w8235
                  disable-tunnel: w8234 -> [w8239 _]
                  frame Disabled {
                    n3185 = Unbundle By Name(w8239) -> ("单体电压过高"=w8238:dbl)
                    n3186 = call "输入分辨率计算-EV05.vi"("1字节?"=FALSE, "数值"=w8238, "偏移量"=0.0, "分辨率"=0.001) -> ("低字节"=w8240:dbl, "高字节1"=w8242:dbl)  [unwired: 1 in, 5 out]
                  }
                  frame Enabled {
                    w8245 = 255 ("高字节1")
                  }
                }
                n3187 = Build Array(w8237, w8235) -> (w8236:i32[])
              }
              frame 8 {
                # "单体电压过低"
                n3188 = disable-structure shown="启用" {
                  disable-tunnel: [w8254 w8257] -> w8249
                  disable-tunnel: [w8252 w8257] -> w8247
                  disable-tunnel: w8246 -> [w8251 _]
                  frame Disabled {
                    n3189 = Unbundle By Name(w8251) -> ("单体电压过低"=w8250:dbl)
                    n3190 = call "输入分辨率计算-EV05.vi"("1字节?"=FALSE, "数值"=w8250, "偏移量"=0.0, "分辨率"=0.001) -> ("低字节"=w8252:dbl, "高字节1"=w8254:dbl)  [unwired: 1 in, 5 out]
                  }
                  frame Enabled {
                    w8257 = 255 ("高字节1")
                  }
                }
                n3191 = Build Array(w8249, w8247) -> (w8248:i32[])
              }
              frame 9 {
                # "充电电流过高"
                n3192 = disable-structure shown="启用" {
                  disable-tunnel: [w8266 w8269] -> w8261
                  disable-tunnel: [w8264 w8269] -> w8259
                  disable-tunnel: w8258 -> [w8263 _]
                  frame Disabled {
                    n3193 = Unbundle By Name(w8263) -> ("充电电流过高"=w8262:dbl)
                    n3194 = call "输入分辨率计算-EV05.vi"("1字节?"=FALSE, "数值"=w8262, "偏移量"=-3000.0, "分辨率"=0.1) -> ("低字节"=w8264:dbl, "高字节1"=w8266:dbl)  [unwired: 1 in, 5 out]
                  }
                  frame Enabled {
                    w8269 = 255 ("高字节1")
                  }
                }
                n3195 = Build Array(w8261, w8259) -> (w8260:i32[])
              }
              frame 10 {
                # "放电电流过高"
                n3196 = disable-structure shown="启用" {
                  disable-tunnel: [w8278 w8281] -> w8273
                  disable-tunnel: [w8276 w8281] -> w8271
                  disable-tunnel: w8270 -> [w8275 _]
                  frame Enabled {
                    n3197 = Unbundle By Name(w8275) -> ("放电电流过高"=w8274:dbl)
                    n3198 = call "输入分辨率计算-EV05.vi"("1字节?"=FALSE, "数值"=w8274, "偏移量"=0.0, "分辨率"=0.1) -> ("低字节"=w8276:dbl, "高字节1"=w8278:dbl)  [unwired: 1 in, 5 out]
                  }
                  frame Disabled {
                    w8281 = 255 ("高字节1")
                  }
                }
